vi "Copy_API_Description.vi"(1 "Event":T1, 2 "Input Sequence":cluster{string, string[], dbl[], dbl}[](array[cluster])) -> (0 "Output Sequence":cluster{string, string[], dbl[], dbl}[](array[cluster]))   [LabVIEW 2011]
doc: "This VI copies the API description of the current event to all other events with a matching API ID in the given sequence."
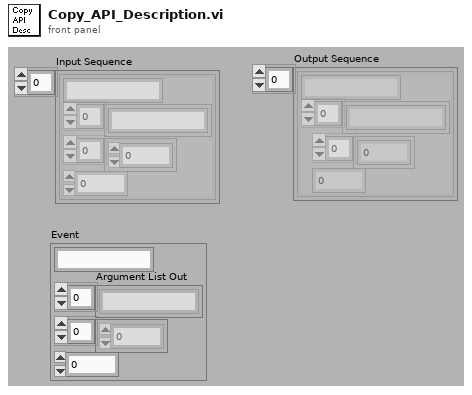
[diagram p1: front panel]
types:
  T1 = cluster{string, "Argument List Out":string[], dbl[], dbl}
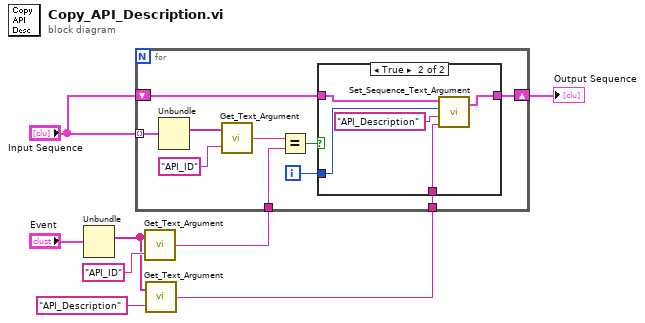
[diagram p0: block diagram]
diagram:
  n1 = Unbundle("Event") -> ("Argument List Out"=w4:string[])  [unwired: 3 out]
  n2 = call "Get_Text_Argument.vi"("Argument"="API_ID", "Argument List"=w4) -> ("Text"=w6:string)
  n3 = call "Get_Text_Argument.vi"("Argument"="API_Description", "Argument List"=w4) -> ("Text"=w2:string)
  n4 = for {
    tunnel: w6 -> [w15]
    tunnel: "Input Sequence" -> [w14] mode=indexing
    shift-right: [w11] -> w1
    shift-left: "Input Sequence" -> [w12]
    tunnel: w2 -> [w9]
    i -> [w10]
    n5 = Unbundle(w14) -> (w18:string[])  [unwired: 3 out]
    n6 = call "Get_Text_Argument.vi"("Argument"="API_ID", "Argument List"=w18) -> ("Text"=w16:string)
    n7 = Equal?(x=w16, y=w15) -> (x = y?=w13:bool)
    n8 = case shown="True" w13 {
      tunnel: w12 -> [w19 w23]
      tunnel: [w19 w20] -> w11
      tunnel: w10 -> [_ w24]
      tunnel: w9 -> [_ w21]
      frame False {
      }
      frame True {
        n9 = call "Set_Sequence_Text_Argument.vi"("Text"=w21, "Argument"="API_Description", "Index"=w24, "Input Sequence"=w23) -> ("Output Sequence"=w20:cluster{string, string[], dbl[], dbl}[])  [unwired: 1 out]
      }
    }
  }
  "Output Sequence" <- w1
